vi "lab 4-1.vi"() -> ()   [LabVIEW 2021]
panel:
  out "Array 4":dbl[](array[numeric])
  out "Array 3":dbl[](array[numeric])
  out "Array 2":dbl[](array[numeric])
  out "vr: relative uncartainty value (%)":dbl
  out "v :absulate uncartainty":dbl
  out "si :experimental waste":dbl
  out "Array":dbl[](array[numeric])
  out "R : best estimated measurement":dbl
  out "sum":dbl
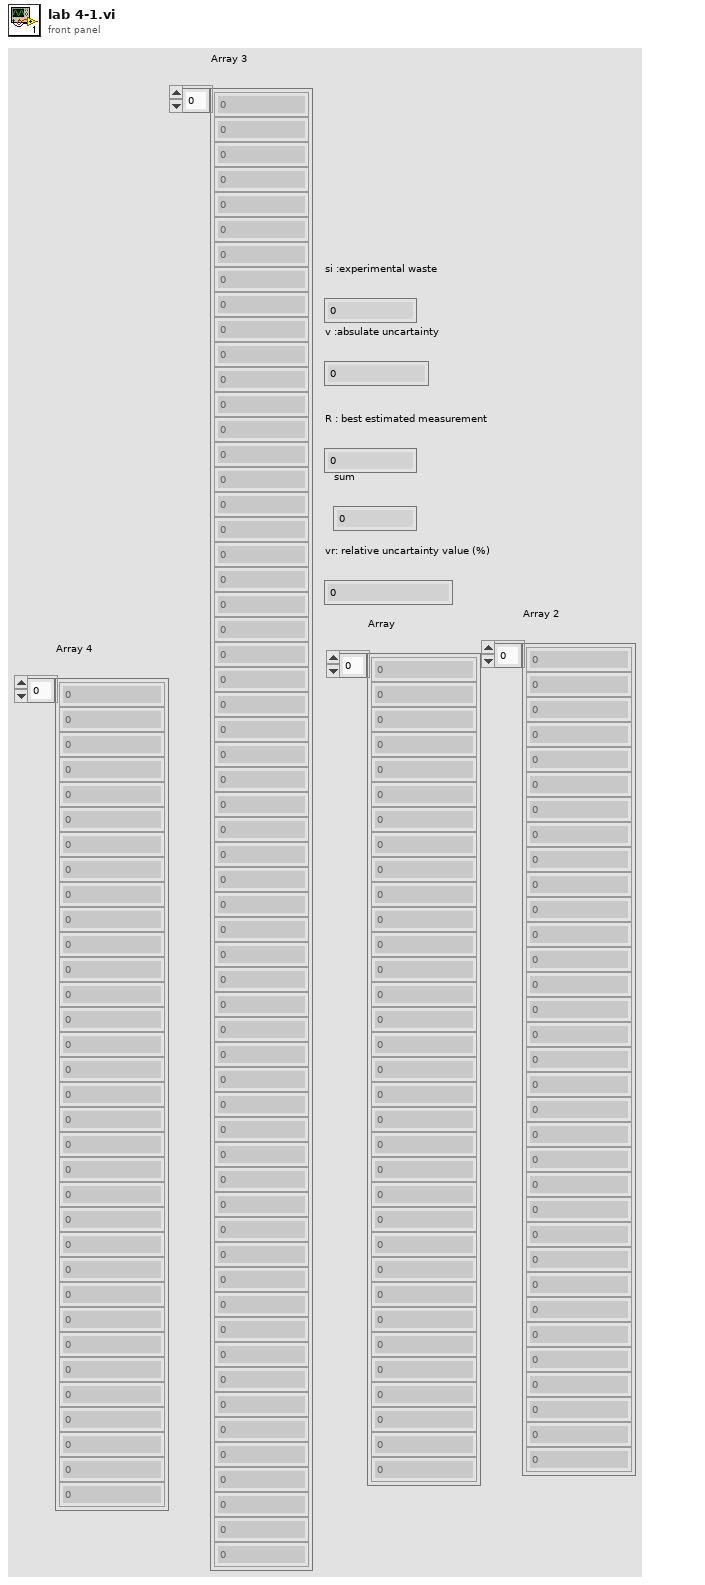
[diagram p1: front panel]
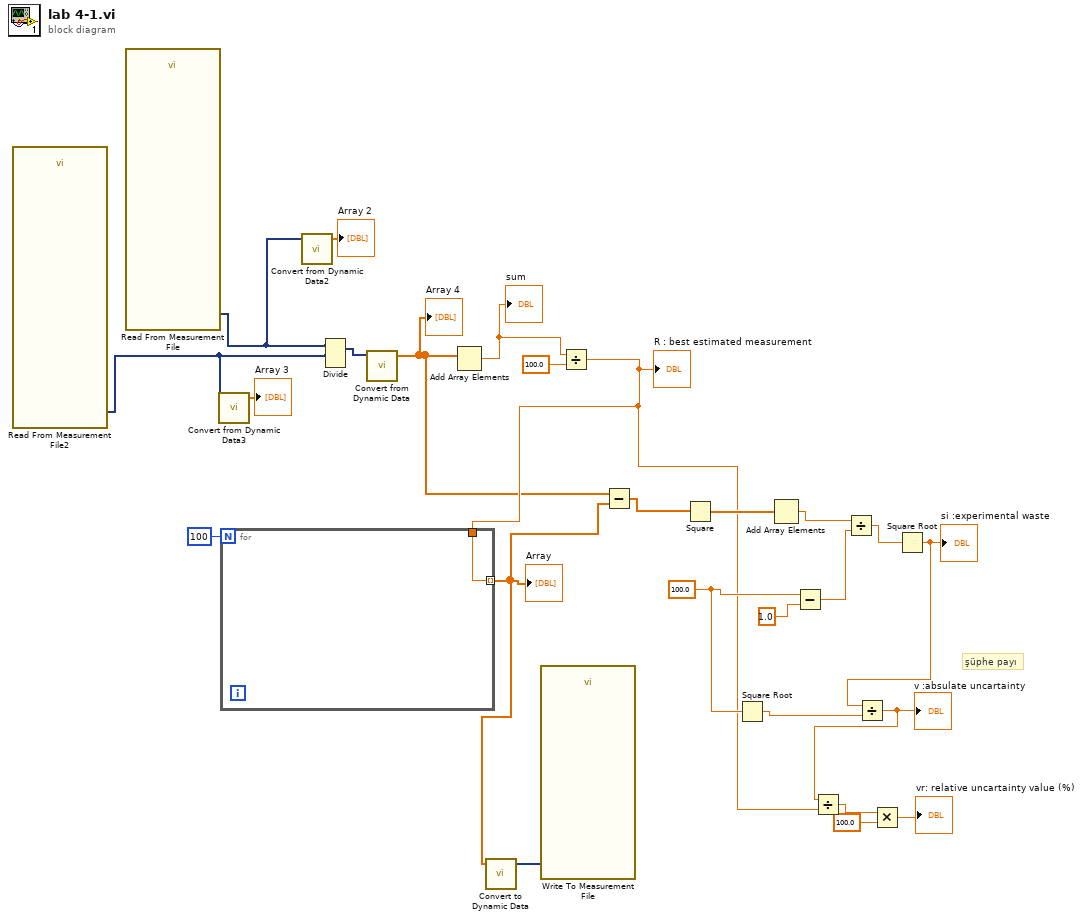
[diagram p0: block diagram]
diagram:
  w14 = 100.0 ("x")
  # "şüphe payı"
  n1 = call "Read From Measurement File2"() -> ("Signals"=w3:dynamicdata)  [unwired: 6 in, 5 out]
  n2 = call "Read From Measurement File"() -> ("Signals"=w4:dynamicdata)  [unwired: 6 in, 5 out]
  n3 = call "Convert from Dynamic Data3"("Dynamic Data Type"=w3) -> ("Array"=→"Array 3":dbl[])  [unwired: 3 in]
  n4 = call "Convert from Dynamic Data2"("Dynamic Data Type"=w4) -> ("Array"=→"Array 2":dbl[])  [unwired: 3 in]
  n5 = Divide(1:w3, 2:w4) -> (0:w2:dynamicdata)  [unwired: 1 in, 1 out]
  n6 = call "Convert from Dynamic Data"("Dynamic Data Type"=w2) -> ("Array"=w1:dbl[])  [unwired: 3 in]
  "Array 4" <- w1
  n7 = Add Array Elements(numeric array=w1) -> (sum=w25:dbl)
  "sum" <- w25
  n8 = Divide(x=w25, y=100.0) -> (x/y=w10:dbl)
  "R : best estimated measurement" <- w10
  n9 = for {
    N: 100 -> [_]
    tunnel: w10 -> [w26]
    tunnel: [w26] -> w21 mode=indexing
  }
  "Array" <- w21
  n10 = call "Convert to Dynamic Data"("Waveform"=w21) -> ("Dynamic Data Type"=w22:dynamicdata)  [unwired: 3 in]
  n11 = call "Write To Measurement File"("Signals"=w22) -> ()  [unwired: 16 in, 3 out]
  n12 = Subtract(x=w1, y=w21) -> (x-y=w20:dbl[])
  n13 = Square(x=w20) -> (x^2=w19:dbl[])
  n14 = Square Root(x=w14) -> (sqrt(x)=w12:dbl)
  n15 = Add Array Elements(numeric array=w19) -> (sum=w17:dbl)
  n16 = Subtract(x=w14, y=1.0) -> (x-y=w16:dbl)
  n17 = Divide(x=w17, y=w16) -> (x/y=w15:dbl)
  n18 = Square Root(x=w15) -> (sqrt(x)=w13:dbl)
  "si :experimental waste" <- w13
  n19 = Divide(x=w13, y=w12) -> (x/y=w11:dbl)
  "v :absulate uncartainty" <- w11
  n20 = Divide(x=w11, y=w10) -> (x/y=w9:dbl)
  n21 = Multiply(x=w9, y=100.0) -> (x*y=→"vr: relative uncartainty value (%)":dbl)
